vi "Open FP.vi"(8 "error in":errorcluster, 9 "Open FP":bool, 10 "Selected VIs":string[](array[string]), 11 "Application in":refnum<vi>) -> (0 "error out":errorcluster)   [LabVIEW 2013, in "LVTM.lvlib"]
uses:
  LVTM.lvlib
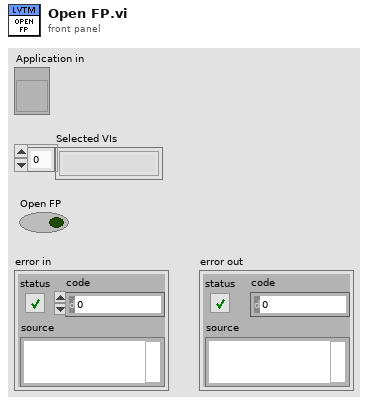
[diagram p1: front panel]
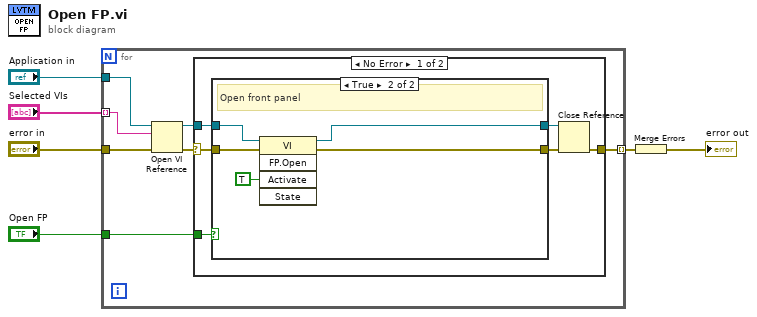
[diagram p0: block diagram]
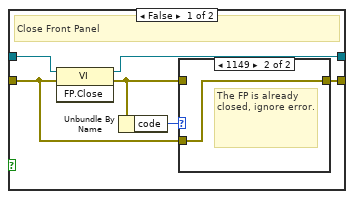
[diagram p2: hidden frame]
diagram:
  n1 = for {
    tunnel: [w13] -> w2 mode=indexing
    tunnel: "error in" -> [w12]
    tunnel: "Selected VIs" -> [w11] mode=indexing
    tunnel: "Application in" -> [w10]
    tunnel: "Open FP" -> [w8]
    n2 = Open VI Reference(application reference (local)=w10, vi path=w11, error in (no error)=w12) -> (vi reference=w9:refnum<vi>, error out=w7:errorcluster)  [unwired: 3 out]
    n3 = case shown="No Error" w7 {
      selector: w7 -> [w14 _]
      tunnel: [w19 _] -> w13
      tunnel: w9 -> [w17 _]
      tunnel: w8 -> [w15 _]
      frame No Error {
        n4 = case shown="True" w15 {
          tunnel: w14 -> [w20 w31]
          tunnel: [w21 w30] -> w18
          tunnel: w17 -> [w25 w29]
          tunnel: [w24 w28] -> w16
          frame False {
            # "Close Front Panel"
            n5 = invoke class="VI" method="FP.Close"(reference=w25, error in=w20) -> (reference out=w24:refnum<vi>, error out=w22:errorcluster)  [unwired: 1 in, 1 out]
            n6 = Unbundle By Name(w22) -> ("code"=w23:i32)
            n7 = case shown="1149" w23 {
              tunnel: w22 -> [w26 _]
              tunnel: [w26 w27] -> w21
              tunnel: w20 -> [_ w27]
              frame 0, Default {
              }
              frame 1149 {
                # "The FP is already closed, ignore error."
              }
            }
          }
          frame True {
            # "Open front panel"
            n8 = invoke class="VI" method="FP.Open"(reference=w29, error in=w31, "Activate"=TRUE ("Activate?")) -> (reference out=w28:refnum<vi>, error out=w30:errorcluster)  [unwired: 2 in, 3 out]
          }
        }
        n9 = Close Reference(reference=w16, error in (no error)=w18) -> (error out=w19:errorcluster)
      }
      frame Error {
        # "This VI is no longer in the memory"
      }
    }
  }
  n10 = Merge Errors(w2) -> (→"error out":errorcluster)
